vi "Getattribute.vi"(8 "error in (no error)":errorcluster, 11 "OneOfTemplate in":refnum<class "nidaqmx_grpc_GetTaskAttributeStringRequest_attribute_enum.lvclass">) -> (0 "error out":errorcluster, 2 "Get_Val":T1, 3 "OneOfTemplate out":refnum<class "nidaqmx_grpc_GetTaskAttributeStringRequest_attribute_enum.lvclass">)   [LabVIEW 2021, in "NI DAQmx_server.lvlib" / "nidaqmx_grpc_GetTaskAttributeStringRequest_attribute_enum.lvclass"]
uses:
  nidaqmx_grpc_GetTaskAttributeStringRequest_attribute_enum.lvclass
  nidaqmx_grpc_TaskStringAttribute.ctl
  nidaqmx_grpc_GetTaskAttributeStringRequest_attribute_enum.lvclass/nidaqmx_grpc_GetTaskAttributeStringRequest_attribute_enum.ctl
  NI DAQmx_server.lvlib
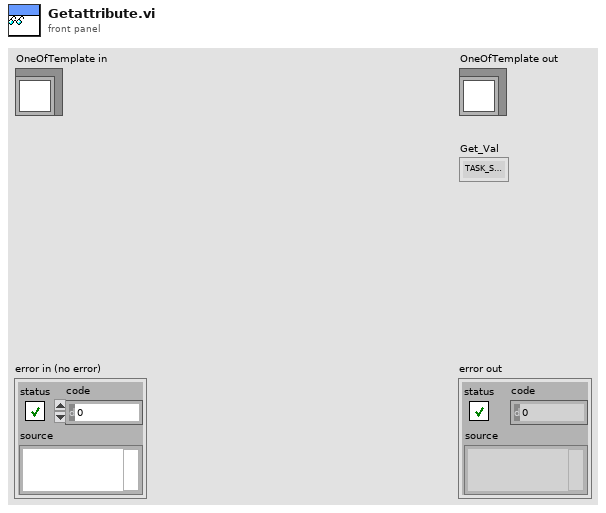
[diagram p1: front panel]
types:
  T1 = typedef "NI DAQmx_server.lvlib/nidaqmx_grpc_TaskStringAttribute.ctl" = enum32{"TASK_STRING_ATTRIBUTE_UNSPECIFIED", "TASK_ATTRIBUTE_CHANNELS", "TASK_ATTRIBUTE_NAME", "TASK_ATTRIBUTE_DEVICES"}
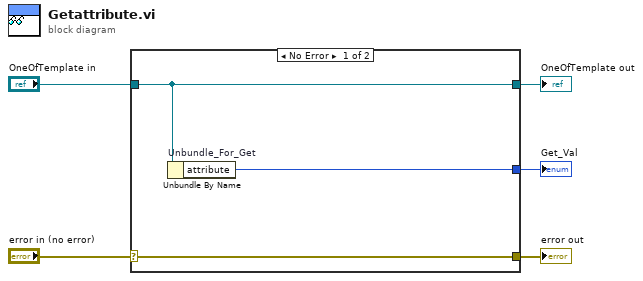
[diagram p0: block diagram]
diagram:
  n1 = case shown="No Error" "error in (no error)" {
    selector: "error in (no error)" -> [w8 w9]
    tunnel: [w8 w9] -> w4
    tunnel: [w7 w10] -> w2
    tunnel: "OneOfTemplate in" -> [w7 w10]
    tunnel: [w6 _] -> w1
    frame No Error {
      n2 = Unbundle By Name "Unbundle_For_Get"(w7) -> ("attribute"=w6:T1)
    }
    frame Error {
    }
  }
  "error out" <- w4
  "OneOfTemplate out" <- w2
  "Get_Val" <- w1
